vi "Common-IsBetween.vi"(9 "比例(0.1)":dbl=0.1, 10 "基数":dbl, 11 "x":dbl) -> (3 "范围内？":bool)   [LabVIEW 2014]
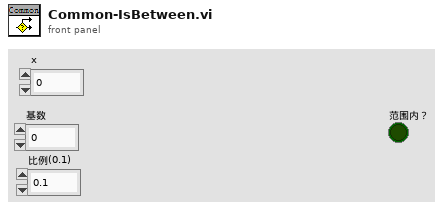
[diagram p1: front panel]
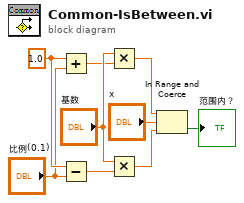
[diagram p0: block diagram]
diagram:
  w5 = 1.0 ("x")
  n1 = Add(x=w5, y="比例(0.1)") -> (x+y=w6:dbl)
  n2 = Subtract(x=w5, y="比例(0.1)") -> (x-y=w3:dbl)
  n3 = Multiply(x="基数", y=w6) -> (x*y=w1:dbl)
  n4 = Multiply(x="基数", y=w3) -> (x*y=w2:dbl)
  n5 = In Range and Coerce(upper limit=w1, x="x", lower limit=w2) -> (In Range?=→"范围内？":bool)  [unwired: 1 out]
